vi "Position Telemetry Button.vi"(8 "Error In":errorcluster, 11 "Telem":refnum<vi>) -> (0 "Error Out":errorcluster)   [LabVIEW 2014]
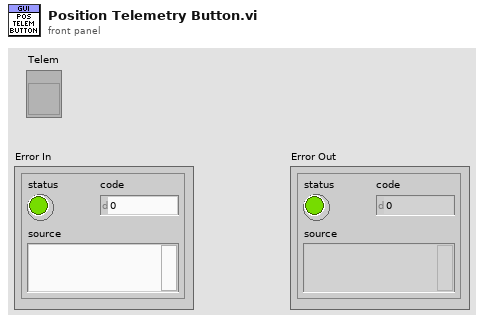
[diagram p1: front panel]
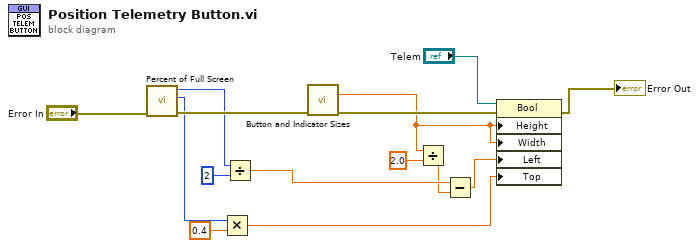
[diagram p0: block diagram]
diagram:
  n1 = call "Percent of Full Screen.vi"("error in (no error)"="Error In") -> ("error out"=w14:errorcluster, "Bottom"=w5:i16, "Right"=w10:i16)  [unwired: 8 in]
  n2 = Multiply(x=w5, y=0.4) -> (x*y=w3:dbl)
  n3 = Divide(x=w10, y=i16 2) -> (x/y=w8:dbl)
  n4 = call "Button and Indicator Sizes.vi"("error in (no error)"=w14) -> ("Button Height"=w12:dbl, "error out"=w13:errorcluster)  [unwired: 10 in, 3 out]
  n5 = Divide(x=w12, y=2.0) -> (x/y=w7:dbl)
  n6 = Subtract(x=w8, y=w7) -> (x-y=w6:dbl)
  n7 = property class="Bool"(reference="Telem", error in=w13, "Height"=w12, "Width"=w12, "Left"=w6, "Top"=w3) -> (error out=→"Error Out":errorcluster)  [unwired: 1 out]
